vi "SP Calculate TXY.vi"(10 "SP Array (SXX, SXY, SYX, SYY)":cdb[](array[numeric])) -> (2 "TXY":cdb)   [LabVIEW 2011]
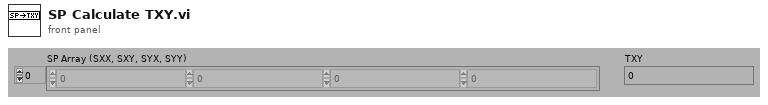
[diagram p1: front panel]
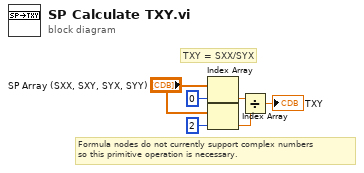
[diagram p0: block diagram]
diagram:
  # "TXY = SXX/SYX"
  # "Formula nodes do not currently support complex numbers\nso this primitive operation is necessary."
  n1 = Index Array(array="SP Array (SXX, SXY, SYX, SYY)", index=0) -> (element=w3:cdb)
  n2 = Index Array(array="SP Array (SXX, SXY, SYX, SYY)", index=2) -> (element=w2:cdb)
  n3 = Divide(x=w3, y=w2) -> (x/y=→"TXY":cdb)
